vi "TrapezoidalAcceleration.vi"(8 "MaxMotorChangeBackward":dbl, 9 "MaxMotorChangeForward":dbl, 10 "Desired":dbl, 11 "Actual":dbl) -> (2 "In range?":bool, 3 "New Actual":dbl)   [LabVIEW 2015]
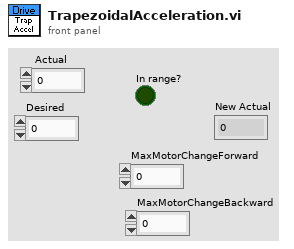
[diagram p1: front panel]
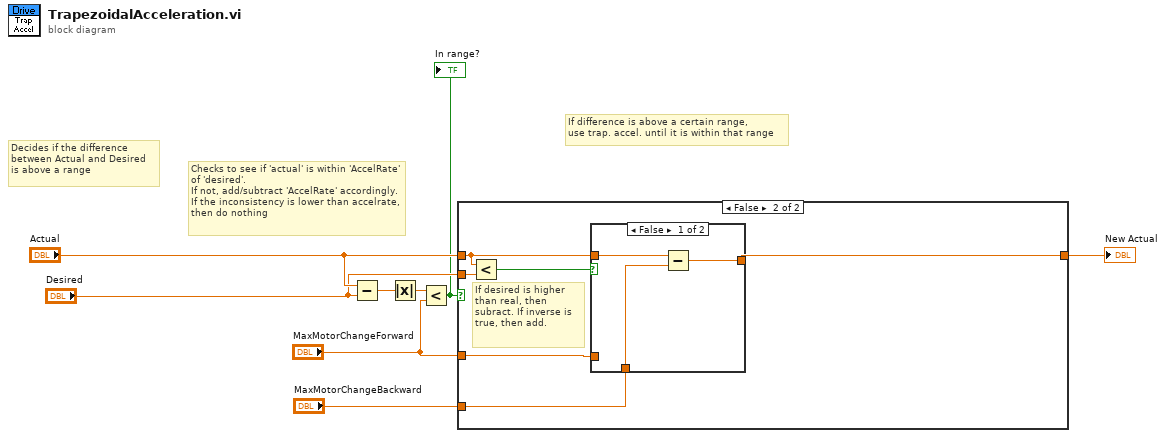
[diagram p0: block diagram]
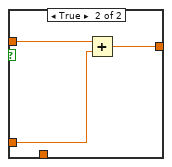
[diagram p3: hidden frame]
diagram:
  # "If difference is above a certain range,\nuse trap. accel. until it is within that range"
  # "Checks to see if 'actual' is within 'AccelRate' of 'desired'.\nIf not, add/subtract 'AccelRate' accordingly. If the inconsistency is lower than accelrate, then do nothing"
  # "Decides if the difference\nbetween Actual and Desired\nis above a range"
  n1 = Subtract(x="Actual", y="Desired") -> (x-y=w4:dbl)
  n2 = Absolute Value(x=w4) -> (abs(x)=w5:dbl)
  n3 = Less?(x=w5, y="MaxMotorChangeForward") -> (x < y?=w3:bool)
  "In range?" <- w3
  n4 = case shown="False" w3 {
    tunnel: [w9 w15] -> w8
    tunnel: "Actual" -> [_ w14]
    tunnel: "Desired" -> [w9 w12]
    tunnel: "MaxMotorChangeForward" -> [_ w11]
    tunnel: "MaxMotorChangeBackward" -> [_ w10]
    frame True {
    }
    frame False {
      # "If desired is higher than real, then subract. If inverse is true, then add."
      n5 = Less?(x=w14, y=w12) -> (x < y?=w13:bool)
      n6 = case shown="False" w13 {
        tunnel: w14 -> [w17 w20]
        tunnel: [w18 w21] -> w15
        tunnel: w11 -> [_ w19]
        tunnel: w10 -> [w16 _]
        frame False {
          n7 = Subtract(x=w17, y=w16) -> (x-y=w18:dbl)
        }
        frame True {
          n8 = Add(x=w20, y=w19) -> (x+y=w21:dbl)
        }
      }
    }
  }
  "New Actual" <- w8
